vi "Read ResultList.vi"(8 "error in (no error)":errorcluster, 11 "Execution in":refnum<class "Execution.lvclass">) -> (0 "error out":errorcluster, 2 "ResultList":T1[](array[typedef]), 3 "Execution out":refnum<class "Execution.lvclass">)   [LabVIEW 2015, in "Execution.lvclass"]
uses:
  Execution.lvclass
  STEP_RESULT.ctl
  Step.lvclass
  Step/STEP_STATUS.ctl
  STEP_MEASURE_RESULT.ctl
  Step/OUTPUT_DATA_TYPE.ctl
  OutputUI/OUTPUT_CHECK_TYPE.ctl
  Execution.lvclass/Execution.ctl
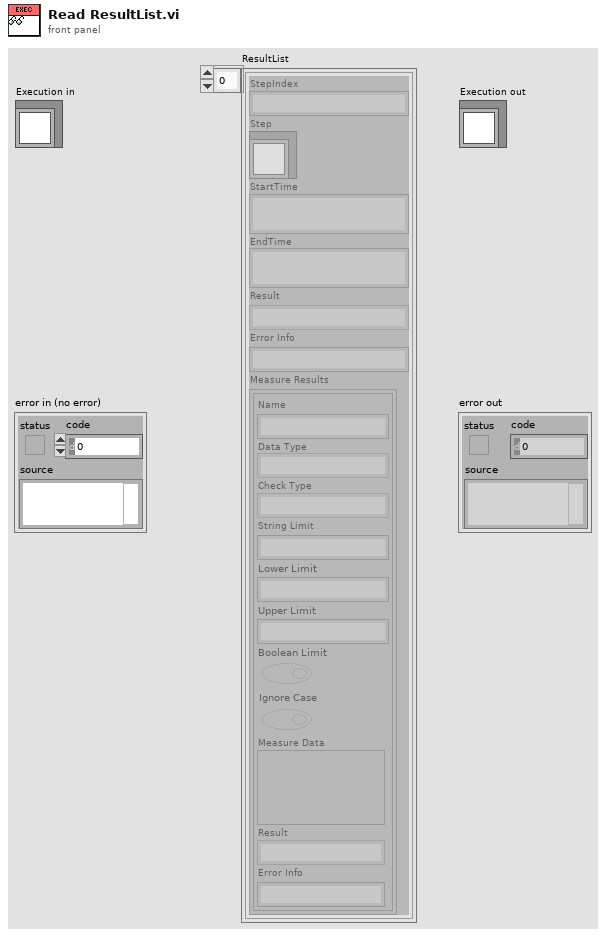
[diagram p1: front panel]
types:
  T1 = typedef "Execution.lvclass/STEP_RESULT.ctl" = cluster{"StepIndex":u32, "Step":refnum<class "Step.lvclass">, "StartTime":timestamp, "EndTime":timestamp, "Result":T2, "Error Info":string, "Measure Results":T3[]}
  T2 = typedef "Step.lvclass/STEP_STATUS.ctl" = enum16{"Skipped", "Done", "Passed", "Failed", "Error"}
  T3 = typedef "Execution.lvclass/STEP_MEASURE_RESULT.ctl" = cluster{"Name":string, "Data Type":T4, "Check Type":T5, "String Limit":string, "Lower Limit":dbl, "Upper Limit":dbl, "Boolean Limit":bool, "Ignore Case":bool, "Measure Data":variant, "Result":T2, "Error Info":string}
  T4 = typedef "Step.lvclass/OUTPUT_DATA_TYPE.ctl" = enum16{"Boolean", "String", "Numeric", "Other"}
  T5 = typedef "Step.lvclass/OUTPUT_CHECK_TYPE.ctl" = enum16{"INVALID", "DO_NOT_CHECK", "RECORD", "VARIABLE", "EQUAL", "NOT_EQUAL", "STR_CONTAINS", "STR_START_WITH", "STR_END_WITH", "STR_REGEX_MATCH", "NUM_GT", "NUM_LT", "NUM_GE", "NUM_LE", "NUM_RANGE", "NUM_RANGE_BDY"}
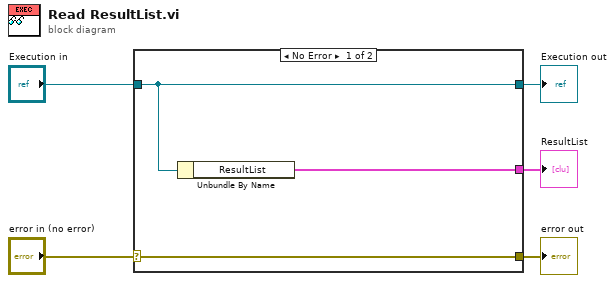
[diagram p0: block diagram]
diagram:
  n1 = case shown="No Error" "error in (no error)" {
    selector: "error in (no error)" -> [w8 w9]
    tunnel: [w8 w9] -> w4
    tunnel: [w7 w10] -> w2
    tunnel: "Execution in" -> [w7 w10]
    tunnel: [w6 _] -> w1
    frame No Error {
      n2 = Unbundle By Name(w7) -> ("ResultList"=w6:T1[])
    }
    frame Error {
    }
  }
  "error out" <- w4
  "Execution out" <- w2
  "ResultList" <- w1
